vi "Get Bits.vi"(8 "error in (no error)":errorcluster, 10 "Count (1)":i32=1, 11 "Packet in":refnum<class "Packet.lvclass">) -> (0 "error out":errorcluster, 2 "Bits":bool[](array[boolean]), 3 "Packet out":refnum<class "Packet.lvclass">)   [LabVIEW 2020, in "Packet.lvclass"]
uses:
  Packet.lvclass
  Packet.lvclass/Packet.ctl
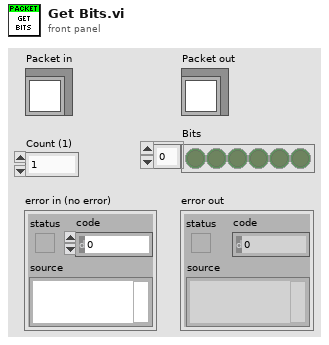
[diagram p1: front panel]
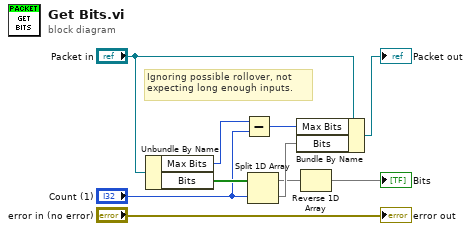
[diagram p0: block diagram]
diagram:
  # "Ignoring possible rollover, not expecting long enough inputs."
  n1 = Unbundle By Name("Packet in") -> ("Max Bits"=w8:i32, "Bits"=w5:bool[])
  n2 = Subtract(x=w8, y="Count (1)") -> (x-y=w9:i32)
  n3 = Split 1D Array(array=w5, index="Count (1)") -> (first subarray=w2:bool[], second subarray=w3:bool[])
  n4 = Bundle By Name(cluster="Packet in", "Max Bits"=w9, "Bits"=w3) -> (→"Packet out":refnum<class "Packet.lvclass">)
  n5 = Reverse 1D Array(array=w2) -> (reversed array=→"Bits":bool[])
  "error out" <- "error in (no error)"
